vi "Start Cycle.vi"(8 "error in (no error)":errorcluster, 11 "State Machine in":refnum<class "State Machine.lvclass">) -> (0 "error out":errorcluster, 3 "State Machine out":refnum<class "State Machine.lvclass">)   [LabVIEW 2024, in "State Machine.lvlib" / "State Machine.lvclass"]
uses:
  State Machine.lvclass
  State Machine.lvclass/State Machine.ctl
  State/State/State.lvclass
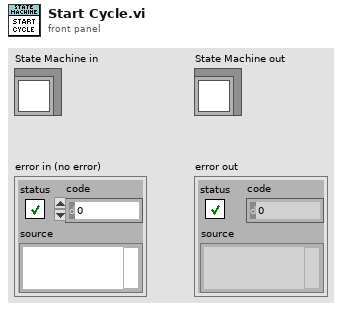
[diagram p1: front panel]
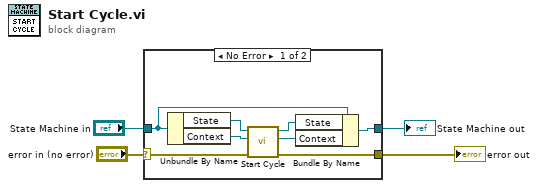
[diagram p0: block diagram]
diagram:
  n1 = case shown="No Error" "error in (no error)" {
    selector: "error in (no error)" -> [w7 w14]
    tunnel: [w6 w14] -> w3
    tunnel: [w10 w13] -> w1
    tunnel: "State Machine in" -> [w11 w13]
    frame No Error {
      n2 = Unbundle By Name(w11) -> ("State"=w5:refnum<class "State.lvclass">, "Context"=w12:refnum<data-value>)
      n3 = call-dynamic "Start Cycle.vi"("error in (no error)"=w7, "Context in"=w12, "State in"=w5) -> ("error out"=w6:errorcluster, "Context out"=w8:refnum<data-value>, "State out"=w9:refnum<class "State.lvclass">)  [unwired: 6 in]
      n4 = Bundle By Name(cluster=w11, "State"=w9, "Context"=w8) -> (w10:refnum<class "State Machine.lvclass">)
    }
    frame Error {
    }
  }
  "error out" <- w3
  "State Machine out" <- w1
